vi "FPGA_ADC.vi"() -> ()   [LabVIEW 2013]
uses:
  <vilib>/Platform/TimedLoop/XDataNode/timing_clust.ctl
  <vilib>/Platform/TimedLoop/XDataNode/nitl_modes.ctl
  <vilib>/Platform/TimedLoop/XDataNode/wakeup.ctl
  <vilib>/rvi/Emulation/niFpgaSctlEmulationGetInTimedLoop.vi
  <vilib>/rvi/Emulation/niFpgaEmulationReportErrorSimple.vi
  <vilib>/rvi/Emulation/niFpgaGetClockAttributes.vi
  <vilib>/rvi/FIFO/Fifo_Resource/nirvififoEmulationReadFpgaImpl.vi
  <vilib>/rvi/DataTransferAndStorage/Container/Common/niFpgaContainerGetUniqueNameForEmu.vi
  <vilib>/rvi/Emulation/niFpgaProcessEmulError.vi
  <vilib>/rvi/Emulation/niFpgaCriticalErrorInLSC.vi
  <vilib>/rvi/FIFO/Fifo_Resource/nirvififoEmulationWriteFpgaImpl.vi
  <vilib>/rvi/FIFO/Fifo_Resource/nirvififoEmulationClearFpgaImpl.vi
  <vilib>/rvi/eio/common/nirviEmuTemplateMethod_errors.vi
  <vilib>/rvi/FIFO/Fifo_Resource/nirvififoEmulationGetNumberOfElementsToReadFpgaImpl.vi
  <vilib>/rvi/interface/RandomDataEmulation/nirviRandomDataFPGAFIFO.vi
  <vilib>/rvi/interface/RandomDataEmulation/niFpgaRandomDataHandleErrors.vi
  <vilib>/rvi/Memory/Memory_Emulation/nirvimemoryFastEmulationFpgaImpl.vi
  <instcachedir>/0/nirvimemoryFastEmulationFpgaImpl_5FBAB50466BC4C939F684F8805638BFC.lvgen/nirvimemoryFastEmulationFpgaImpl_5FBAB50466BC4C939F684F8805638BFC_001.vi
  <vilib>/rvi/Memory/Memory_Emulation/nirvimemoryFastEmulation.vi
  <vilib>/rvi/Memory/Memory_Emulation/nirvimemoryEmulation.vi
  <vilib>/rvi/DataTransferAndStorage/Container/XNode/niFpgaContainer.xnode
  <vilib>/rvi/FIFO/Fifo_Resource/nirvififoEmulationRead.vi
  <vilib>/rvi/FIFO/Fifo_Resource/nirvififoEmulationWrite.vi
  <vilib>/rvi/FIFO/Fifo_Resource/nirvififoEmulationClear.vi
  <vilib>/eio/EIOMethodNode/EIOMethodNode.xnode
  <vilib>/rvi/FIFO/Fifo_Resource/nirvififoEmulationGetNumberOfElementsToRead.vi
  <vilib>/eio/EIONode/EIONode.xnode
  <vilib>/Platform/TimedLoop/XDataNode/XDataNode.xnode
  <vilib>/rvi/interface/RandomDataEmulation/nirviRandomDataFpgaReadWriteTemplate.vi
  <vilib>/Platform/TimedLoop/XDataNode/XDNodeRunTimeDep.lvlib
panel:
  in  "get order":bool
  in  "order in":u64=434597364041252864
  in  "trig mode":enum8{"ramp", "RT"}(ring)=enum."RT"
  in  "Npts to read":u16=100
  out "i meas":i32
  in  "meas ON":bool
  out "i trig detect":i32=18739822
  in  "trig input":u8
  in  "trig edge":enum8{"falling", "rising", "both"}(ring)=enum."both"
  out "trig detected":bool
  in  "trig resets":i32
  in  "manual trig":bool
  in  "trig detect ON":bool
  out "i avg":i32=8 format="%^.3e"
  out "avg timed out 2":bool
  out "avg timed out 1":bool
  out "avg elmt":fxp<+/-,26,5>=-0.0050678253173828125
  out "DMA buffer space":u32=1009
  in  "avg ON":bool
  out "temp buffer elmts":u32=16389
  in  "Navg":u16=1000
  out "i clock":i32=1351237135
  in  "clock divider":u32=40000
  in  "clock ON":bool
  out "i acqu":i32=229444 format="%^.3e"
  in  "Configurations":u16[](array[numeric])=[10296, 10552, 0, 0, 0, 0, 0, 0, 0, 0, 0, 0, 0, 0, 0, 0, 0, 0, 0, 0, 0, 0, 0, 0, 0, 0, 0, 0, 0, 0, 0, 0]
  out "acq timed out":bool
  out "Data [i]":fxp<+/-,26,5>=-0.0050678253173828125
  in  "Nchannels":u8=2
  in  "acqu ON":bool
  out "clock tick":bool
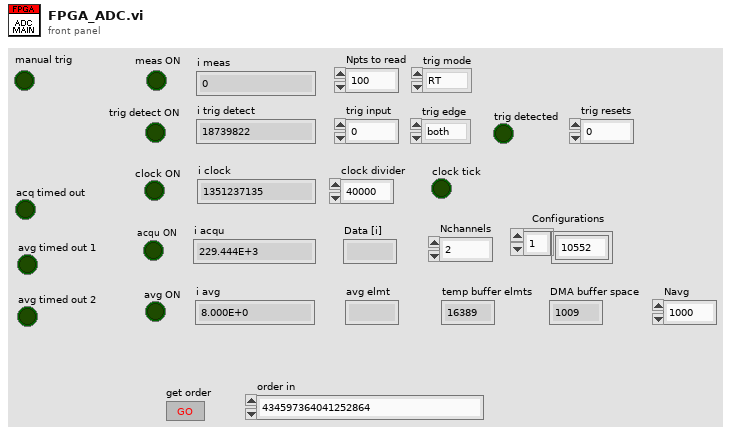
[diagram p1: front panel]
types:
  T1 = typedef "XDNodeRunTimeDep.lvlib/timing_clust.ctl" = cluster{"Expected End [f-1]":u64, "Actual End [f-1]":u64, "Finished Late? [f-1]":bool, "Expected End [i-1]":u64, "Actual End [i-1]":u64, "Finished Late? [i-1]":bool, "Expected Start [i]":u64, "Actual Start [i]":u64, "Expected Start [f]":u64, "Actual Start [f]":u64, "Source Name":string, "Structure Name":string, "Period":i64, "Deadline":i64, "Offset":i64, "Start":i64, "Priority":i32, "Timeout":i32, "Mode":T2, "Wakeup Reason":T3, "Error":errorcluster, "Source Type":string, "Secondary Source Type":string, "Global End Time":u64, "Global Start Time":u64, "Frame Duration":u64, "Iteration Duration":u64, "Assigned CPU":i32, "I/O Scan Engine Mode":u32}
  T2 = typedef "XDNodeRunTimeDep.lvlib/nitl_modes.ctl" = enum32{"No Change", "Process missed periods, maintain original phase", "Discard missed periods, maintain original phase", "Process missed periods, ignore original phase", "Discard missed periods, ignore original phase"}
  T3 = typedef "XDNodeRunTimeDep.lvlib/wakeup.ctl" = enum32{"Normal", "Aborted", "Asynchronous wakeup", "Timing source error", "Timed loop error", "Timeout"}
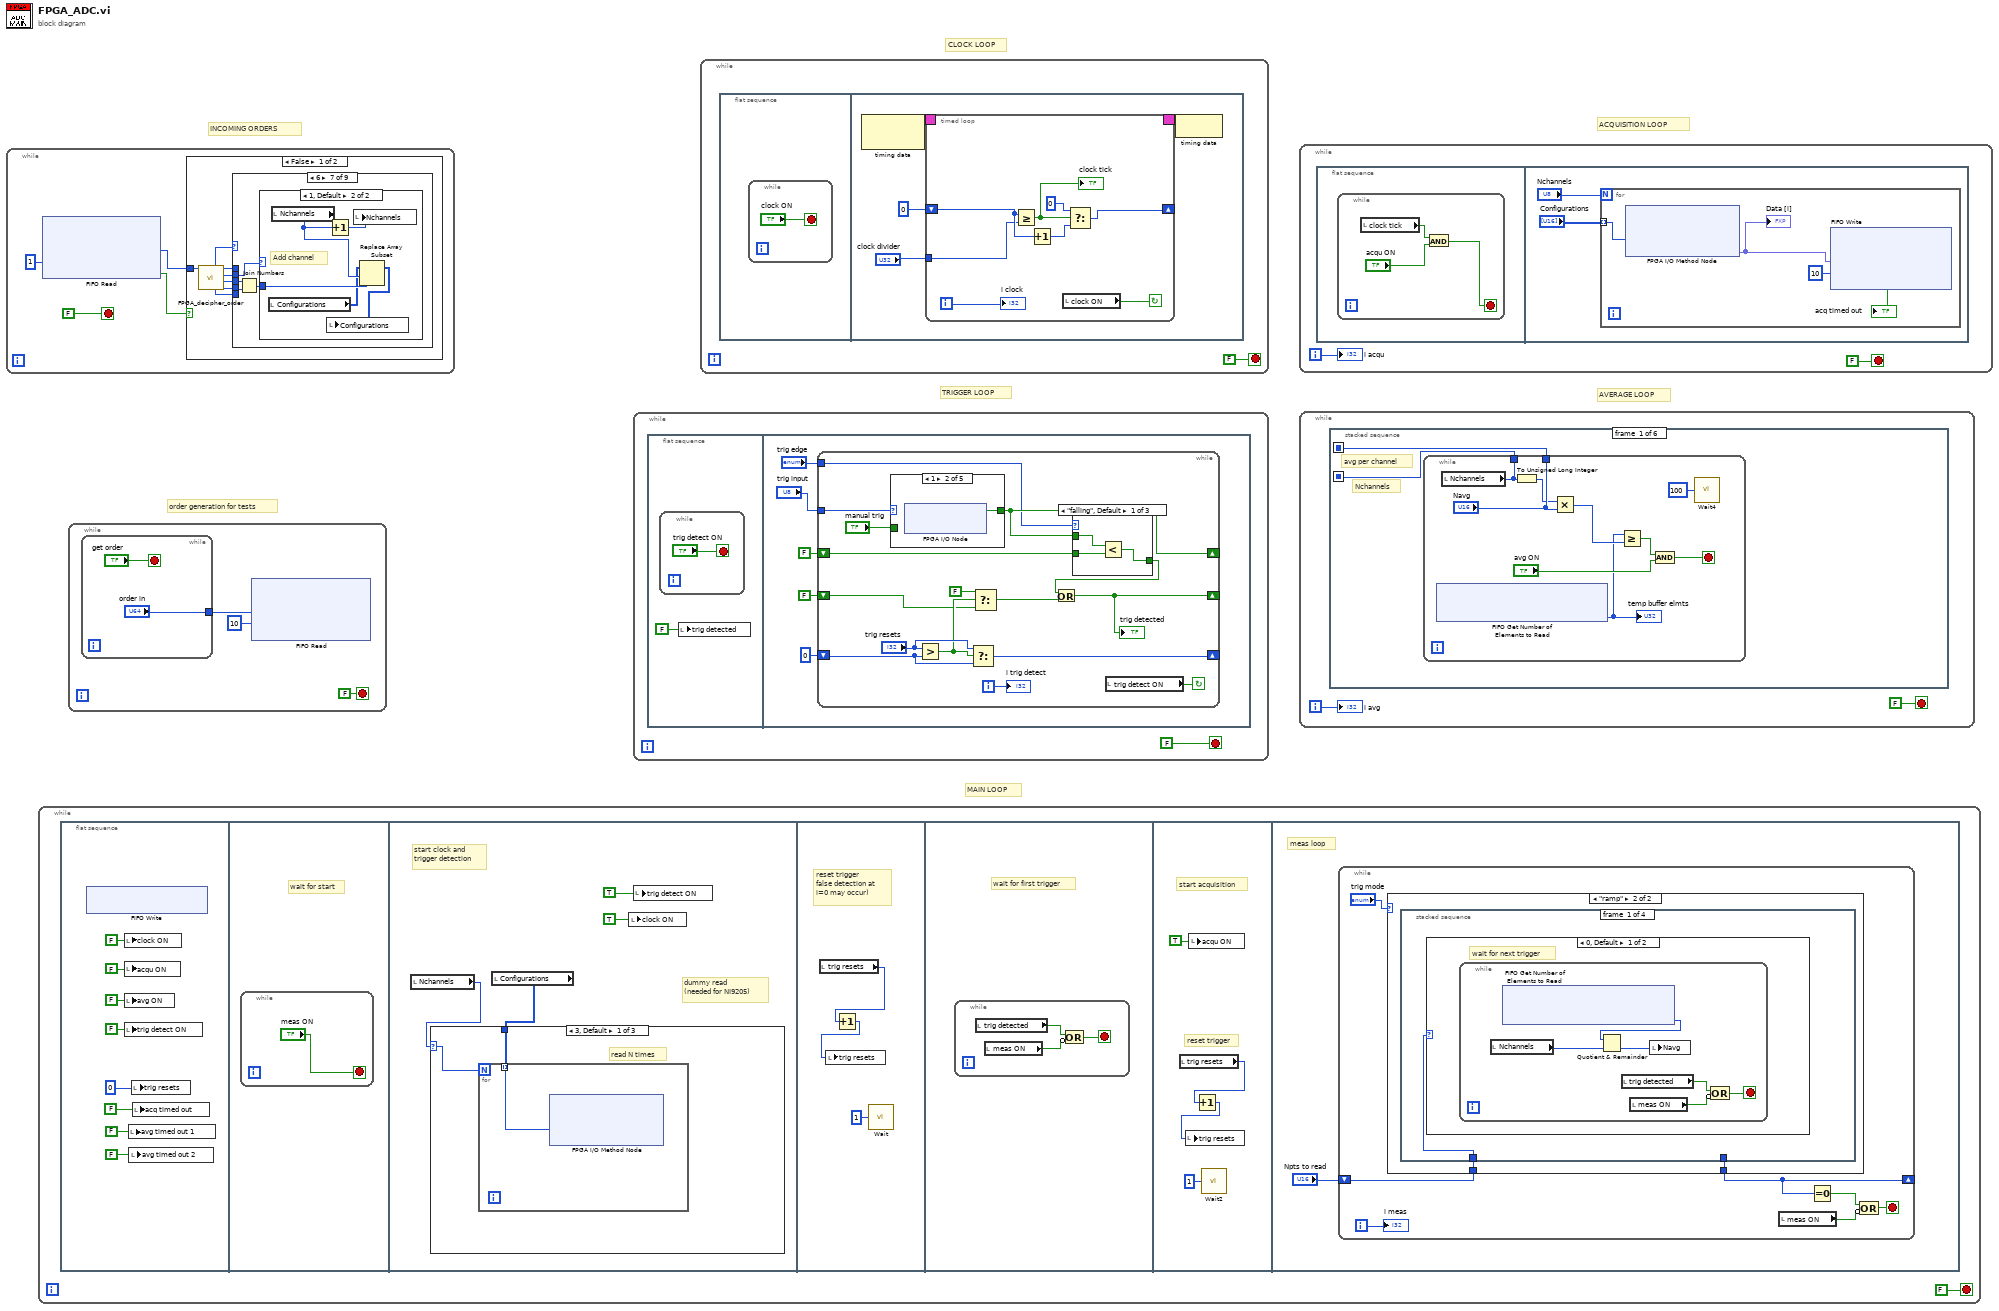
[diagram p0: block diagram]
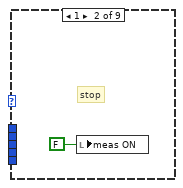
[diagram p3: hidden frame]
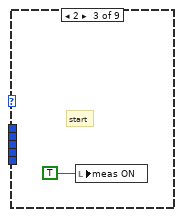
[diagram p4: hidden frame]
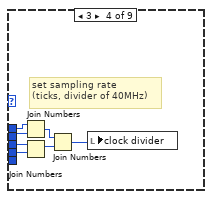
[diagram p5: hidden frame]
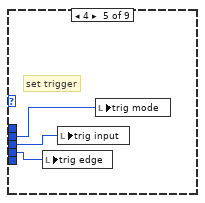
[diagram p6: hidden frame]
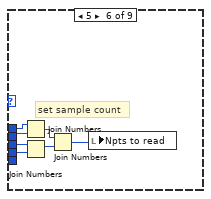
[diagram p7: hidden frame]
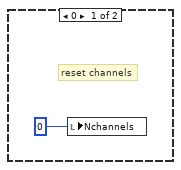
[diagram p8: hidden frame]
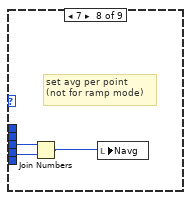
[diagram p9: hidden frame]
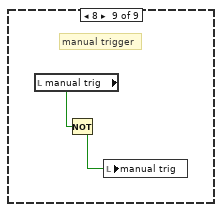
[diagram p10: hidden frame]
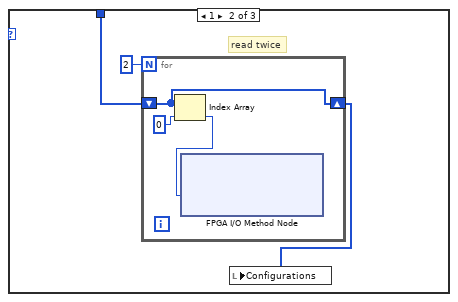
[diagram p12: hidden frame]
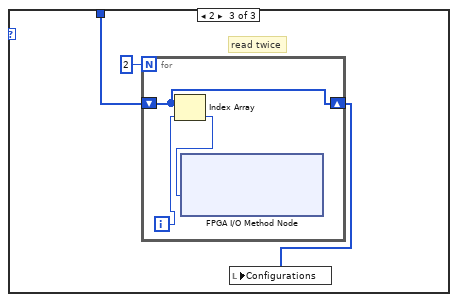
[diagram p13: hidden frame]
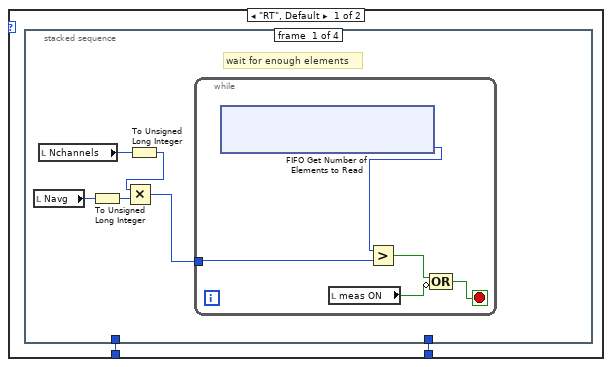
[diagram p14: hidden frame]
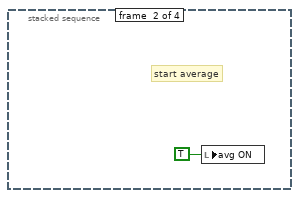
[diagram p15: hidden frame]
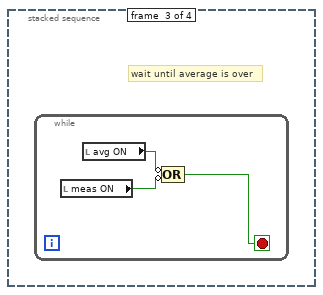
[diagram p16: hidden frame]
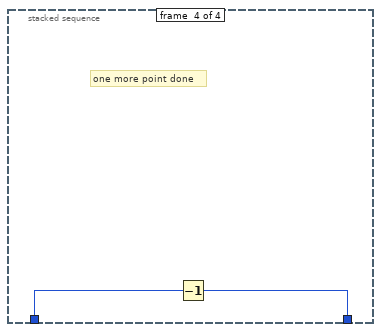
[diagram p17: hidden frame]
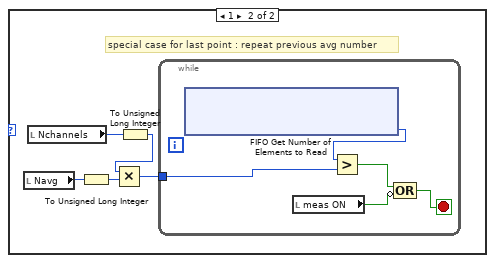
[diagram p18: hidden frame]
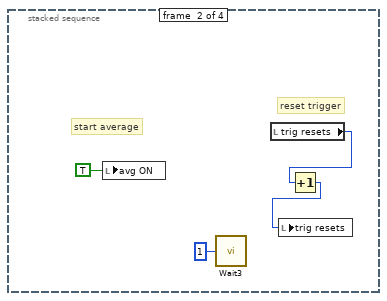
[diagram p19: hidden frame]
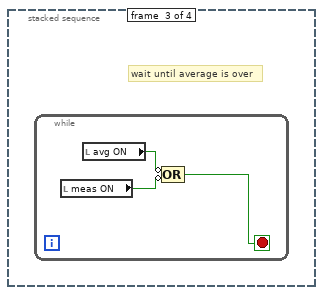
[diagram p20: hidden frame]
diagram:
  # "INCOMING ORDERS"
  # "order generation for tests"
  # "CLOCK LOOP"
  # "TRIGGER LOOP"
  # "AVERAGE LOOP"
  # "MAIN LOOP"
  # "ACQUISITION LOOP"
  n1 = while {
    stop <- FALSE stop-if-true
    n2 = xnode ("FIFO Read")("Timeout"=1) -> ("Element"=w3:u64, "Timed Out?"=w1:bool)  [unwired: 1 in, 1 out]
    n3 = case shown="False" w1 {
      tunnel: w3 -> [w5 _]
      frame False {
        n4 = call "FPGA_decipher_order.vi"("order in"=w5) -> ("data 1"=w10:u8, "data 2"=w9:u8, "data 3"=w7:u8, "data 4"=w8:u8, "RFU 2"=w6:u8, "order out"=w11:u8)  [unwired: 5 out]
        n5 = case shown="6" w11 {
          tunnel: w10 -> [_ _ _ w19 w23 w29 w33 w42 _]
          tunnel: w9 -> [_ _ _ w20 w21 w30 w34 w43 _]
          tunnel: w8 -> [_ _ _ w18 _ w28 _ _ _]
          tunnel: w7 -> [_ _ _ w17 w22 w27 w31 _ _]
          tunnel: w6 -> [_ _ _ _ _ _ _ _ _]
          frame 0, Default {
          }
          frame 1 {
            # "stop"
            n6 = local write "meas ON"(FALSE ("Stop seq")) -> ()
          }
          frame 2 {
            # "start"
            n7 = local write "meas ON"(TRUE ("Stop seq")) -> ()
          }
          frame 3 {
            # "set sampling rate \n(ticks, divider of 40MHz)"
            n8 = Join Numbers(hi=w18, lo=w17) -> ((hi.lo)=w16:u16)
            n9 = Join Numbers(hi=w20, lo=w19) -> ((hi.lo)=w15:u16)
            n10 = Join Numbers(hi=w16, lo=w15) -> ((hi.lo)=w14:u32)
            n11 = local write "clock divider"(w14) -> ()
          }
          frame 4 {
            # "set trigger"
            n12 = local write "trig edge"(w23) -> ()
            n13 = local write "trig input"(w21) -> ()
            n14 = local write "trig mode"(w22) -> ()
          }
          frame 5 {
            # "set sample count"
            n15 = Join Numbers(hi=w28, lo=w27) -> ((hi.lo)=w26:u16)
            n16 = Join Numbers(hi=w30, lo=w29) -> ((hi.lo)=w25:u16)
            n17 = Join Numbers(hi=w26, lo=w25) -> ((hi.lo)=w24:u32)
            n18 = local write "Npts to read"(w24) -> ()
          }
          frame 6 {
            n19 = Join Numbers(hi=w34, lo=w33) -> ((hi.lo)=w32:u16)
            n20 = case shown="1, Default" w31 {
              tunnel: w32 -> [_ w39]
              frame 0 {
                # "reset channels"
                n21 = local write "Nchannels"(u8 0 ("Nchannels")) -> ()
              }
              frame 1, Default {
                # "Add channel"
                n22 = local read "Configurations"() -> (w37:u16[])
                n23 = local read "Nchannels"() -> (w38:u8)
                n24 = Increment(x=w38) -> (x+1=w40:u8)
                n25 = local write "Nchannels"(w40) -> ()
                n26 = Replace Array Subset(array=w37, new element=w39, index=w38) -> (w36:u16[])
                n27 = local write "Configurations"(w36) -> ()
              }
            }
          }
          frame 7 {
            # "set avg per point\n(not for ramp mode)"
            n28 = Join Numbers(hi=w43, lo=w42) -> ((hi.lo)=w41:u16)
            n29 = local write "Navg"(w41) -> ()
          }
          frame 8 {
            # "manual trigger"
            n30 = local read "manual trig"() -> (w45:bool)
            n31 = Not(x=w45) -> (.not. x?=w44:bool)
            n32 = local write "manual trig"(w44) -> ()
          }
        }
      }
      frame True {
      }
    }
  }
  n33 = while {
    stop <- FALSE stop-if-true
    n34 = flat-sequence {
      frame #0 {
        n35 = xnode ("FIFO Write")() -> ()  [unwired: 1 in, 1 out]
        n36 = local write "clock ON"(FALSE ("clock ON")) -> ()
        n37 = local write "acqu ON"(FALSE ("clock ON")) -> ()
        n38 = local write "avg ON"(FALSE ("clock ON")) -> ()
        n39 = local write "trig detect ON"(FALSE ("clock ON")) -> ()
        n40 = local write "avg timed out 1"(FALSE ("clock ON")) -> ()
        n41 = local write "avg timed out 2"(FALSE ("clock ON")) -> ()
        n42 = local write "trig resets"(0 ("trig resets")) -> ()
        n43 = local write "acq timed out"(FALSE ("clock ON")) -> ()
      }
      frame #1 {
        # "wait for start"
        n44 = while {
          stop <- "meas ON" stop-if-true
        }
      }
      frame #2 {
        # "dummy read\n(needed for NI9205)"
        # "start clock and\ntrigger detection"
        n45 = local read "Nchannels"() -> (w57:u8)
        n46 = local read "Configurations"() -> (w56:u16[])
        n47 = case shown="3, Default" w57 {
          selector: w57 -> [w61 _ _]
          tunnel: w56 -> [w60 w63 w70]
          frame 3, Default {
            # "read N times"
            n48 = for {
              N: w61 -> [_]
              tunnel: w60 -> [w62] mode=indexing
              n49 = xnode "FPGA I/O Method Node"("Configuration [i+2]"=w62) -> ()  [unwired: 2 in, 3 out]
            }
          }
          frame 1 {
            # "read twice"
            n50 = for {
              N: 2 -> [_]
              shift-right: [w66] -> w65
              shift-left: w63 -> [w66]
              n51 = Index Array(array=w66, index=0) -> (element=w67:u16)
              n52 = xnode "FPGA I/O Method Node"("Configuration [i+2]"=w67) -> ()  [unwired: 2 in, 3 out]
            }
            n53 = local write "Configurations"(w65) -> ()
          }
          frame 2 {
            # "read twice"
            n54 = for {
              N: 2 -> [_]
              shift-right: [w73] -> w71
              shift-left: w70 -> [w73]
              i -> [w72]
              n55 = Index Array(array=w73, index=w72) -> (element=w74:u16)
              n56 = xnode "FPGA I/O Method Node"("Configuration [i+2]"=w74) -> ()  [unwired: 2 in, 3 out]
            }
            n57 = local write "Configurations"(w71) -> ()
          }
        }
        n58 = local write "clock ON"(TRUE ("meas ON")) -> ()
        n59 = local write "trig detect ON"(TRUE ("meas ON")) -> ()
      }
      frame #3 {
        # "reset trigger \nfalse detection at \ni=0 may occur)"
        n60 = local read "trig resets"() -> (w77:i32)
        n61 = Increment(x=w77) -> (x+1=w76:i32)
        n62 = local write "trig resets"(w76) -> ()
        n63 = call "Wait"("Count(uSec)"=u32 1) -> ()  [unwired: 1 out]
      }
      frame #4 {
        # "wait for first trigger"
        n64 = while {
          stop <- w78 stop-if-true
          n65 = local read "trig detected"() -> (w79:bool)
          n66 = local read "meas ON"() -> (w80:bool)
          n67 = Compound Arithmetic op=OR(w79, invert w80) -> (w78:bool)
        }
      }
      frame #5 {
        # "reset trigger"
        # "start acquisition"
        n68 = local read "trig resets"() -> (w82:i32)
        n69 = local write "acqu ON"(TRUE ("acqu ON")) -> ()
        n70 = Increment(x=w82) -> (x+1=w83:i32)
        n71 = local write "trig resets"(w83) -> ()
        n72 = call "Wait2"("Count(uSec)"=u32 1) -> ()  [unwired: 1 out]
      }
      frame #6 {
        # "meas loop"
        n73 = while {
          shift-right: [w87] -> _
          shift-left: "Npts to read" -> [w88]
          i -> [w90]
          stop <- w91 stop-if-true
          n74 = case shown="\"ramp\"" "trig mode" {
            tunnel: w88 -> [w94 w112]
            tunnel: [w93 w111] -> w87
            frame "RT", Default {
              n75 = stacked-sequence {
                tunnel: w94 -> [_ _ _ w109]
                tunnel: [_ _ _ w110] -> w93
                frame #0 {
                  # "wait for enough elements"
                  n76 = local read "Navg"() -> (w95:u16)
                  n77 = local read "Nchannels"() -> (w99:u8)
                  n78 = To Unsigned Long Integer(number=w95) -> (unsigned 32bit integer=w96:u32)
                  n79 = To Unsigned Long Integer(number=w99) -> (unsigned 32bit integer=w98:u32)
                  n80 = Multiply(x=w98, y=w96) -> (x*y=w97:u32)
                  n81 = while {
                    tunnel: w97 -> [w100]
                    stop <- w102 stop-if-true
                    n82 = xnode ("FIFO Get Number of Elements to Read")() -> ("Number of Elements to Read"=w101:u32)  [unwired: 1 in, 1 out]
                    n83 = local read "meas ON"() -> (w103:bool)
                    n84 = Greater?(x=w101, y=w100) -> (0:w104:bool)
                    n85 = Compound Arithmetic op=OR(w104, invert w103) -> (w102:bool)
                  }
                }
                frame #1 {
                  # "start average"
                  n86 = local write "avg ON"(TRUE ("acqu ON")) -> ()
                }
                frame #2 {
                  # "wait until average is over"
                  n87 = while {
                    stop <- w107 stop-if-true
                    n88 = local read "meas ON"() -> (w108:bool)
                    n89 = local read "avg ON"() -> (w106:bool)
                    n90 = Compound Arithmetic op=OR(invert w106, invert w108) -> (w107:bool)
                  }
                }
                frame #3 {
                  # "one more point done"
                  n91 = Decrement(x=w109) -> (x-1=w110:u16)
                }
              }
            }
            frame "ramp" {
              n92 = stacked-sequence {
                tunnel: w112 -> [w113 _ _ w137]
                tunnel: [_ _ _ w138] -> w111
                frame #0 {
                  n93 = case shown="0, Default" w113 {
                    frame 0, Default {
                      # "wait for next trigger"
                      n94 = while {
                        stop <- w117 stop-if-true
                        n95 = local read "Nchannels"() -> (w114:u8)
                        n96 = xnode ("FIFO Get Number of Elements to Read")() -> ("Number of Elements to Read"=w116:u32)  [unwired: 1 in, 1 out]
                        n97 = Quotient & Remainder(x=w116, y=w114) -> (floor(x/y)=w115:u32)  [unwired: 1 out]
                        n98 = local read "trig detected"() -> (w118:bool)
                        n99 = local read "meas ON"() -> (w119:bool)
                        n100 = local write "Navg"(w115) -> ()
                        n101 = Compound Arithmetic op=OR(w118, invert w119) -> (w117:bool)
                      }
                    }
                    frame 1 {
                      # "special case for last point : repeat previous avg number"
                      n102 = local read "Navg"() -> (w120:u16)
                      n103 = local read "Nchannels"() -> (w122:u8)
                      n104 = To Unsigned Long Integer(number=w120) -> (unsigned 32bit integer=w121:u32)
                      n105 = To Unsigned Long Integer(number=w122) -> (unsigned 32bit integer=w123:u32)
                      n106 = Multiply(x=w123, y=w121) -> (x*y=w124:u32)
                      n107 = while {
                        tunnel: w124 -> [w125]
                        stop <- w127 stop-if-true
                        n108 = xnode ("FIFO Get Number of Elements to Read")() -> ("Number of Elements to Read"=w126:u32)  [unwired: 1 in, 1 out]
                        n109 = local read "meas ON"() -> (w128:bool)
                        n110 = Greater?(x=w126, y=w125) -> (0:w129:bool)
                        n111 = Compound Arithmetic op=OR(w129, invert w128) -> (w127:bool)
                      }
                    }
                  }
                }
                frame #1 {
                  # "reset trigger"
                  # "start average"
                  n112 = local write "avg ON"(TRUE ("acqu ON")) -> ()
                  n113 = call "Wait3"("Count(uSec)"=u32 1) -> ()  [unwired: 1 out]
                  n114 = local read "trig resets"() -> (w132:i32)
                  n115 = Increment(x=w132) -> (x+1=w131:i32)
                  n116 = local write "trig resets"(w131) -> ()
                }
                frame #2 {
                  # "wait until average is over"
                  n117 = while {
                    stop <- w135 stop-if-true
                    n118 = local read "meas ON"() -> (w136:bool)
                    n119 = local read "avg ON"() -> (w134:bool)
                    n120 = Compound Arithmetic op=OR(invert w134, invert w136) -> (w135:bool)
                  }
                }
                frame #3 {
                  # "one more point done"
                  n121 = Decrement(x=w137) -> (x-1=w138:u16)
                }
              }
            }
          }
          n122 = local read "meas ON"() -> (w92:bool)
          n123 = Equal To 0?(x=w87) -> (x = 0?=w89:bool)
          n124 = Compound Arithmetic op=OR(w89, invert w92) -> (w91:bool)
          "i meas" <- w90
        }
      }
    }
  }
  n125 = while {
    stop <- FALSE stop-if-true
    n126 = while {
      tunnel: ["order in"] -> w139
      stop <- "get order" stop-if-true
    }
    n127 = xnode ("FIFO Read")("Element"=w139, "Timeout"=10) -> ()  [unwired: 1 in, 2 out]
  }
  n128 = while {
    stop <- FALSE stop-if-true
    n129 = flat-sequence {
      frame #0 {
        n130 = while {
          stop <- "trig detect ON" stop-if-true
        }
        n131 = local write "trig detected"(FALSE ("trig detect ON")) -> ()
      }
      frame #1 {
        n132 = while {
          shift-right: [w165] -> _
          shift-left: FALSE ("manual trig") -> [w164]
          shift-right: [w154] -> _
          shift-left: FALSE -> [w158]
          shift-right: [w160] -> _
          shift-left: 0 ("trig resets") -> [w162]
          tunnel: "trig input" -> [w153]
          tunnel: "trig edge" -> [w152]
          i -> [w167]
          stop <- w166 continue-if-true
          n133 = case shown="1" w153 {
            tunnel: [w168 w169 w170 w171 w172] -> w165
            tunnel: "manual trig" -> [w168 _ _ _ _]
            frame 0, Default {
            }
            frame 1 {
              n134 = xnode "FPGA I/O Node"() -> ("Port0/DIO1"=w169:bool)  [unwired: 1 in, 1 out]
            }
            frame 2 {
              n135 = xnode "FPGA I/O Node"() -> ("Port0/DIO2"=w170:bool)  [unwired: 1 in, 1 out]
            }
            frame 3 {
              n136 = xnode "FPGA I/O Node"() -> ("Port0/DIO3"=w171:bool)  [unwired: 1 in, 1 out]
            }
            frame 4 {
              n137 = xnode "FPGA I/O Node"() -> ("Port0/DIO4"=w172:bool)  [unwired: 1 in, 1 out]
            }
          }
          n138 = Greater?(x="trig resets", y=w162) -> (0:w159:bool)
          n139 = Select(t="trig resets", s=w159, f=w162) -> (s? t:f=w160:i32)
          n140 = Select(t=FALSE, s=w159, f=w158) -> (s? t:f=w157:bool)
          n141 = case shown="\"falling\", Default" w152 {
            tunnel: w164 -> [w174 w178 w181]
            tunnel: [w173 w177 w180] -> w163
            tunnel: w165 -> [w175 w176 w179]
            frame "falling", Default {
              n142 = Less?(x=w175, y=w174) -> (x < y?=w173:bool)
            }
            frame "rising" {
              n143 = Greater?(x=w176, y=w178) -> (0:w177:bool)
            }
            frame "both" {
              n144 = Not Equal?(x=w179, y=w181) -> (x != y?=w180:bool)
            }
          }
          n145 = Or(x=w163, y=w157) -> (x .or. y?=w154:bool)
          "trig detected" <- w154
          n146 = local read "trig detect ON"() -> (w166:bool)
          "i trig detect" <- w167
        }
      }
    }
  }
  n147 = while {
    stop <- FALSE stop-if-true
    n148 = flat-sequence {
      frame #0 {
        n149 = while {
          stop <- "clock ON" stop-if-true
        }
      }
      frame #1 {
        n150 = node-c288() -> (w187:T1)  [unwired: 1 in]
        n151 = timed-loop {
          timing: w187 -> [_]
          timing-out: [_] -> w186
          shift-right: [w193] -> _
          shift-left: u32 0 -> [w194]
          tunnel: "clock divider" -> [w188]
          i -> [w191]
          stop <- w190 continue-if-true
          n152 = Greater Or Equal?(x=w194, y=w188) -> (x >= y?=w189:bool)
          "clock tick" <- w189
          n153 = Increment(x=w194) -> (x+1=w195:u32)
          n154 = local read "clock ON"() -> (w190:bool)
          n155 = Select(t=u32 0, s=w189, f=w195) -> (s? t:f=w193:u32)
          "i clock" <- w191
        }
        n156 = node-c288(w186) -> ()
      }
    }
  }
  n157 = while {
    i -> [w200]
    stop <- FALSE stop-if-true
    n158 = flat-sequence {
      frame #0 {
        n159 = while {
          stop <- w202 stop-if-true
          n160 = local read "clock tick"() -> (w204:bool)
          n161 = And(x=w204, y="acqu ON") -> (x .and. y?=w202:bool)
        }
      }
      frame #1 {
        n162 = for {
          N: "Nchannels" -> [_]
          tunnel: "Configurations" -> [w207] mode=indexing
          n163 = xnode "FPGA I/O Method Node"("Configuration [i+2]"=w207) -> ("Data [i]"=w208:fxp<+/-,26,5>)  [unwired: 2 in, 2 out]
          "Data [i]" <- w208
          n164 = xnode ("FIFO Write")("Element"=w208, "Timeout"=10) -> ("Timed Out?"=→"acq timed out":bool)  [unwired: 1 in, 1 out]
        }
      }
    }
    "i acqu" <- w200
  }
  n165 = while {
    i -> [w211]
    stop <- FALSE stop-if-true
    n166 = stacked-sequence {
      seq-local: [w214 _ _ _ _ _] -> [_ _ w225 w229 w243 _]
      seq-local: [w213 _ _ _ _ _] -> [_ _ _ w230 w242 _]
      frame #0 {
        # "avg per channel"
        # "Nchannels"
        n167 = while {
          tunnel: ["Navg"] -> w213
          tunnel: [w217] -> w214
          stop <- w222 stop-if-true
          n168 = xnode ("FIFO Get Number of Elements to Read")() -> ("Number of Elements to Read"=w216:u32)  [unwired: 1 in, 1 out]
          "temp buffer elmts" <- w216
          n169 = local read "Nchannels"() -> (w217:u8)
          n170 = To Unsigned Long Integer(number=w217) -> (unsigned 32bit integer=w219:u32)
          n171 = Multiply(x=w219, y="Navg") -> (x*y=w218:u32)
          n172 = Greater Or Equal?(x=w216, y=w218) -> (x >= y?=w221:bool)
          n173 = And(x=w221, y="avg ON") -> (x .and. y?=w222:bool)
          n174 = call "Wait4"("Count(uSec)"=u32 100 ("Count(Ticks)")) -> ()  [unwired: 1 out]
        }
      }
      frame #1 {
        # "avg per channel"
        # "Nchannels"
        n175 = xnode ("FIFO Get Number of Elements to Read")() -> ("Number of Elements to Write"=→"DMA buffer space":u32)  [unwired: 1 in, 1 out]
      }
      frame #2 {
        # "avg per channel"
        # "Nchannels"
        n176 = for {
          N: w225 -> [_]
          i -> [w227]
          n177 = To Unsigned Long Integer(number=w227) -> (unsigned 32bit integer=w226:u32)
          n178 = xnode ("Memory Write")("Address"=w226, "Data"=0) -> ()  [unwired: 1 in, 1 out]
        }
      }
      frame #3 {
        # "avg per channel"
        # "Nchannels"
        n179 = To Long Integer(number=w230) -> (32bit integer=w231:i32)
        n180 = for {
          N: w231 -> [_]
          tunnel: w229 -> [w232]
          n181 = for {
            N: w232 -> [_]
            i -> [w236]
            n182 = xnode ("FIFO Write")("Timeout"=10) -> ("Element"=w233:fxp<+/-,26,5>, "Timed Out?"=→"avg timed out 1":bool)  [unwired: 1 in, 1 out]
            n183 = To Unsigned Long Integer(number=w236) -> (unsigned 32bit integer=w235:u32)
            n184 = xnode ("Memory Read")("Address"=w235) -> ("Data"=w238:i32)  [unwired: 1 in, 1 out]
            n185 = Fixed-Point to Integer Cast(1:w233) -> (0:w234:i32)
            n186 = Add(x=w234, y=w238) -> (x+y=w237:i32)
            n187 = xnode ("Memory Write")("Address"=w235, "Data"=w237) -> ()  [unwired: 1 in, 1 out]
          }
        }
      }
      frame #4 {
        # "avg per channel"
        # "Nchannels"
        n188 = To Long Integer(number=w242) -> (32bit integer=w241:i32)
        n189 = for {
          N: w243 -> [_]
          tunnel: w241 -> [w244]
          i -> [w249]
          n190 = To Unsigned Long Integer(number=w249) -> (unsigned 32bit integer=w248:u32)
          n191 = xnode ("Memory Read")("Address"=w248) -> ("Data"=w246:i32)  [unwired: 1 in, 1 out]
          n192 = Quotient & Remainder(x=w246, y=w244) -> (floor(x/y)=w245:i32)  [unwired: 1 out]
          n193 = Integer to Fixed-Point Cast(fixed-point type=fxp<+/-,26,5> 0.0 ("Element"), integer=w245) -> (fixed-point=w247:fxp<+/-,26,5>)
          "avg elmt" <- w247
          n194 = xnode ("FIFO Write")("Element"=w247, "Timeout"=10) -> ("Timed Out?"=→"avg timed out 2":bool)  [unwired: 1 in, 1 out]
        }
      }
      frame #5 {
        # "avg per channel"
        # "Nchannels"
        n195 = local write "avg ON"(FALSE ("avg ON")) -> ()
      }
    }
    "i avg" <- w211
  }
